vi "Select one Image.vi"(1 "Previous Image (F)":T1, 2 "New Image (T)":T1, 4 "Image to use":bool) -> (6 "Selected Image":T1)   [LabVIEW 2021, in "Image.lvlib"]
uses:
  <vilib>/vision/Image Controls.llb/IMAQ Image.ctl
  Image.lvlib
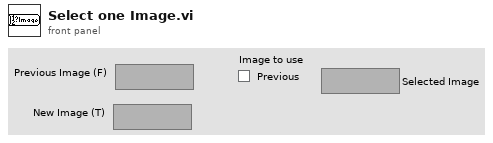
[diagram p1: front panel]
types:
  T1 = typedef "IMAQ Image.ctl" = refnum<image>
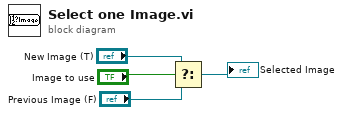
[diagram p0: block diagram]
diagram:
  n1 = Select(t="New Image (T)", s="Image to use", f="Previous Image (F)") -> (s? t:f=→"Selected Image":T1)
